vi "Handle TCP Connection.vi"(4 "Remote Port":u16, 6 "Remote Host":string, 7 "TCPMessageAPI":refnum<class "TCPMessageAPI.lvclass">, 8 "error in (no error)":errorcluster, 9 "Node ID":u32, 10 "Connection State":T1, 11 "TCPConnectionHandler in":refnum<class "TCPConnectionHandler.lvclass">) -> (0 "error out":errorcluster, 3 "TCPConnectionHandler out":refnum<class "TCPConnectionHandler.lvclass">)   [LabVIEW 2020, in "Vecto.lvlib" / "TCPConnectionHandler.lvclass"]
uses:
  TCPConnectionHandler.lvclass
  Connection State.ctl
  TCPMessageService/TCPMessageAPI.lvclass
  Vecto.lvlib
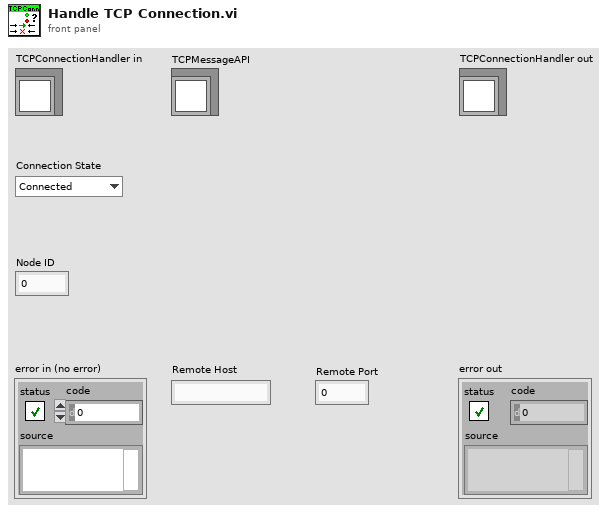
[diagram p1: front panel]
types:
  T1 = typedef "Vecto.lvlib/Connection State.ctl" = enum16{"Connected", "Disconnected"}
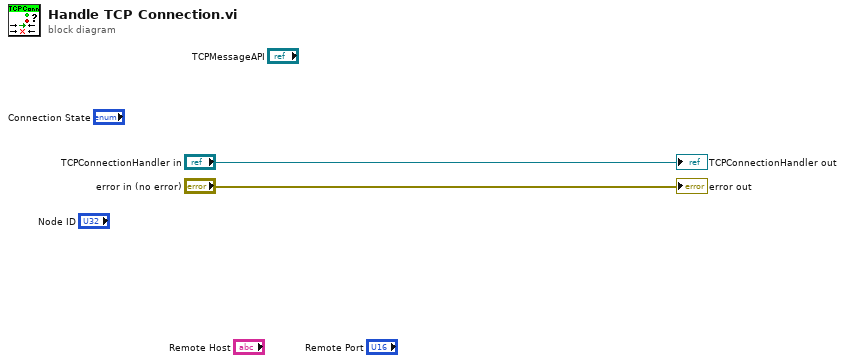
[diagram p0: block diagram]
diagram:
  "error out" <- "error in (no error)"
  "TCPConnectionHandler out" <- "TCPConnectionHandler in"
